vi "DraggingDresser.vi"() -> ()   [LabVIEW 2015]
panel:
  out "Force":dbl[](array[numeric])
  out "Angle for Minimum Force":i32 format="%.1f"
  in  "Coefficient of Kinetic Friction":dbl format="%.1f"
  out "Waveform Graph":dbl[](graph)
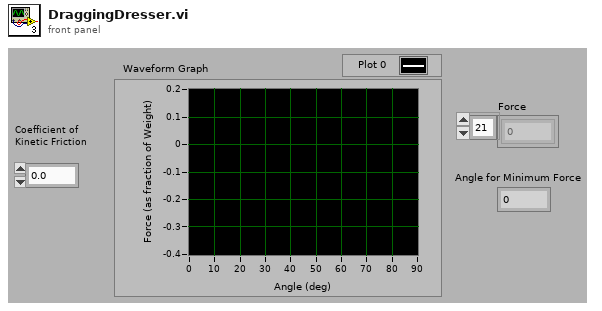
[diagram p1: front panel]
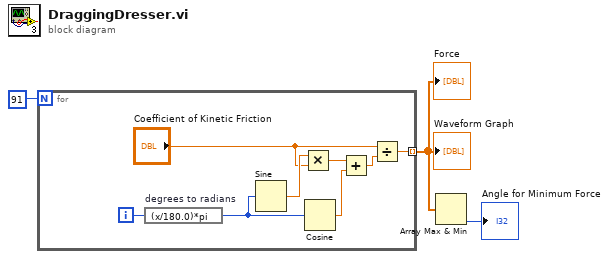
[diagram p0: block diagram]
diagram:
  n1 = for {
    N: 91 -> [_]
    tunnel: [w6] -> w2 mode=indexing
    i -> [w5]
    n2 = expression code="(x/180.0)*pi" "degrees to radians"(w5) -> (w4:i32)
    n3 = Sine(x=w4) -> (sin(x)=w11:dbl)
    n4 = Multiply(x=w11, y="Coefficient of Kinetic Friction") -> (x*y=w8:dbl)
    n5 = Cosine(x=w4) -> (cos(x)=w10:dbl)
    n6 = Add(x=w8, y=w10) -> (x+y=w7:dbl)
    n7 = Divide(x="Coefficient of Kinetic Friction", y=w7) -> (x/y=w6:dbl)
  }
  "Waveform Graph" <- w2
  "Force" <- w2
  n8 = Array Max & Min(array=w2) -> (min index (indices)=→"Angle for Minimum Force":i32)  [unwired: 3 out]
